vi "Mixer Print.vi"(8 "error in (no error)":errorcluster, 10 "On?":bool, 11 "Feeder Actor.lvlib:Mixer.lvclass":refnum<class "Mixer.lvclass">) -> (0 "error out":errorcluster, 3 "Feeder Actor.lvlib:Mixer.lvclass 2":refnum<class "Mixer.lvclass">)   [LabVIEW 2018, in "Feeder Actor.lvlib" / "Mixer.lvclass"]
uses:
  Mixer.lvclass
  C:/Program Files/National Instruments/LabVIEW 2018/vi.lib/ActorFramework/Actor/Actor.lvclass
  <vilib>/ActorFramework/Actor/Actor.lvclass/Actor.ctl
  <vilib>/ActorFramework/Message Enqueuer/Message Enqueuer.lvclass/Message Enqueuer.ctl
  Mixer.lvclass/Mixer.ctl
  <vilib>/ActorFramework/Message Enqueuer/Init from Existing Queue.vi
  <vilib>/ActorFramework/Message Enqueuer/Message Enqueuer.lvclass
  <vilib>/ActorFramework/Actor/Actor.lvclass
  Mixer Messages/Set Mixer Msg/Set Mixer Msg.lvclass
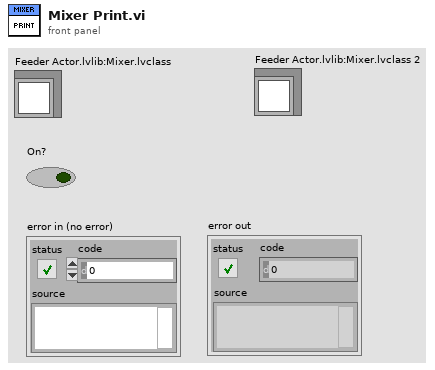
[diagram p1: front panel]
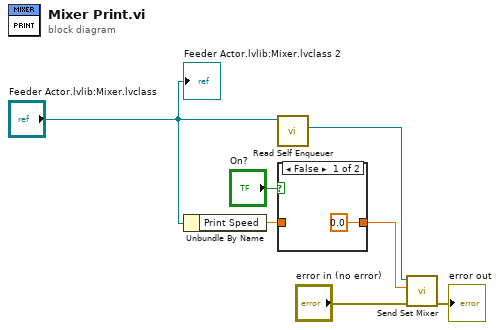
[diagram p0: block diagram]
diagram:
  n1 = Unbundle By Name("Feeder Actor.lvlib:Mixer.lvclass") -> ("Print Speed"=w7:dbl)
  n2 = call <vilib>:"Read Self Enqueuer.vi"("Actor"="Feeder Actor.lvlib:Mixer.lvclass") -> ("Self Enqueuer"=w4:refnum<class "Message Enqueuer.lvclass">)  [unwired: 10 in]
  n3 = case shown="False" "On?" {
    tunnel: w7 -> [_ w9]
    tunnel: [0.0 ("Print Speed") w9] -> w3
    frame False {
    }
    frame True {
    }
  }
  n4 = call "Send Set Mixer.vi"("error in (no error)"="error in (no error)", "Mixer"=w3, "Message Enqueuer in"=w4) -> ("error out"=→"error out":errorcluster)  [unwired: 7 in, 1 out]
  "Feeder Actor.lvlib:Mixer.lvclass 2" <- "Feeder Actor.lvlib:Mixer.lvclass"
